vi "Write Test Name.vi"(8 "error in (no error)":errorcluster, 10 "Test Name":string="Test Name", 11 "Null Adapter in":refnum<class "Null Adapter.lvclass">) -> (0 "error out":errorcluster, 3 "Null Adapter out":refnum<class "Null Adapter.lvclass">)   [LabVIEW 2018, in "Null Adapter.lvlib" / "Null Adapter.lvclass"]
uses:
  Null Adapter.lvclass
  Null Adapter.lvclass/Null Adapter.ctl
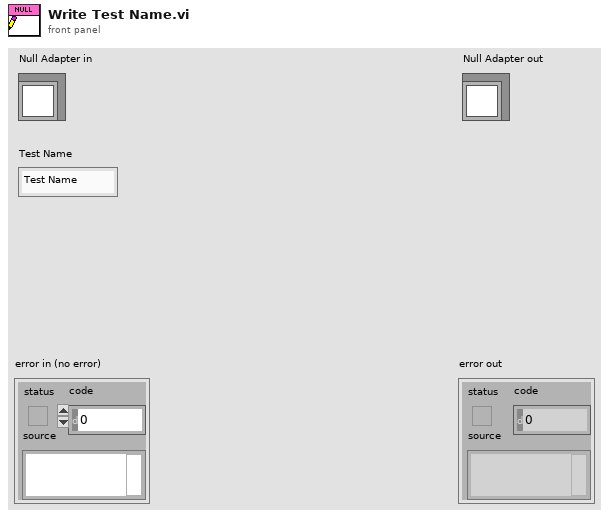
[diagram p1: front panel]
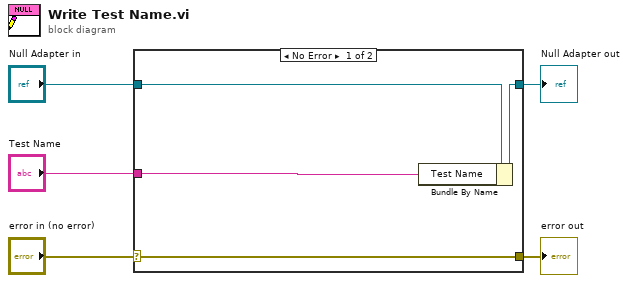
[diagram p0: block diagram]
diagram:
  n1 = case shown="No Error" "error in (no error)" {
    selector: "error in (no error)" -> [w9 w10]
    tunnel: [w9 w10] -> w4
    tunnel: [w7 w11] -> w2
    tunnel: "Null Adapter in" -> [w8 w11]
    tunnel: "Test Name" -> [w6 _]
    frame No Error {
      n2 = Bundle By Name(cluster=w8, "Test Name"=w6) -> (w7:refnum<class "Null Adapter.lvclass">)
    }
    frame Error {
    }
  }
  "error out" <- w4
  "Null Adapter out" <- w2
